vi "Timer Start.vi"(8 "error in (no error)":errorcluster, 10 "Trigger Params":T1, 11 "Instance Name":string) -> (0 "error out":errorcluster, 1 "vi reference":refnum<vi>, 2 "Timer Notifier":refnum<notifier>, 3 "Timer State Rtn event":refnum<user-event>)   [LabVIEW 2015, in "Tool Module.lvlib"]
uses:
  Tool Module.lvlib
  Timer Setup Params Typedef.ctl
  Timer State Return Typedef.ctl
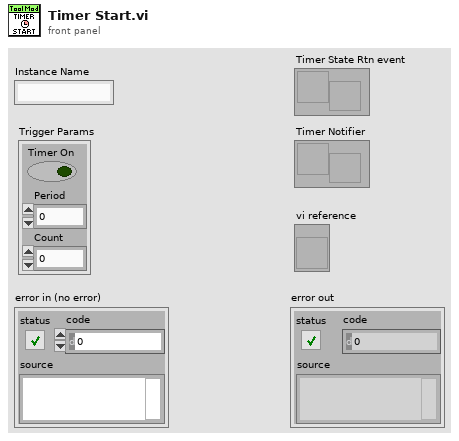
[diagram p1: front panel]
types:
  T1 = typedef "Tool Module.lvlib/Timer Setup Params Typedef.ctl" = cluster{"Timer On":bool, "Period":i32, "Count":i32}
  T2 = typedef "Tool Module.lvlib/Timer State Return Typedef.ctl" = cluster{"Instance Name":string, "On/Off":bool, "Running":bool}
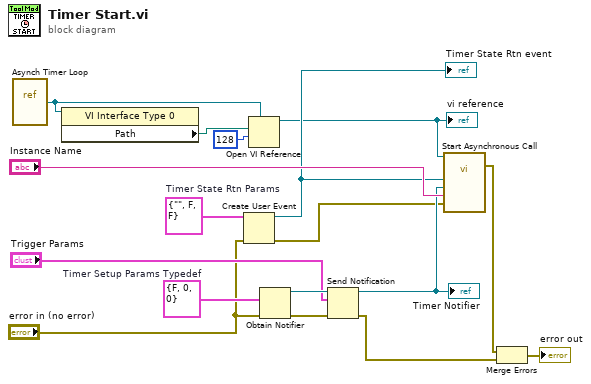
[diagram p0: block diagram]
diagram:
  w7 = T2 {"Instance Name"="", "On/Off"=FALSE, "Running"=FALSE}  # Timer State Rtn Params
  w9 = T1 {"Timer On"=FALSE, "Period"=0, "Count"=0}  # Timer Setup Params Typedef
  n1 = vi-ref "Asynch Timer Loop.vi"() -> (w16:refnum<vi>)
  n2 = property class="VI Interface Type 0"(reference=w16) -> ("Path"=w17:path)  [unwired: 1 in, 2 out]
  n3 = Create User Event(user event datatype=w7, error in="error in (no error)") -> (user event=w6:refnum<user-event>, error out=w8:errorcluster)
  "Timer State Rtn event" <- w6
  n4 = Open VI Reference(type specifier VI Refnum (for type only)=w16, vi path=w17, options=128) -> (vi reference=w1:refnum<vi>)  [unwired: 3 in, 1 out]
  "vi reference" <- w1
  n5 = Obtain Notifier(notification data type=w9, error in (no error)="error in (no error)") -> (notifier out=w14:refnum<notifier>, error out=w13:errorcluster)  [unwired: 2 in, 1 out]
  n6 = Send Notification(notification="Trigger Params", notifier=w14, error in (no error)=w13) -> (notifier out=w11:refnum<notifier>, error out=w5:errorcluster)
  "Timer Notifier" <- w11
  n7 = call-by-ref "Start Asynchronous Call"(reference=w1, "error in (no error)"=w8, "Instance Name"="Instance Name", "Trigger Notifier"=w11, "Trig State Rtn event"=w6) -> (error out=w4:errorcluster)  [unwired: 9 in, 1 out]
  n8 = Merge Errors(w4, w5) -> (→"error out":errorcluster)
